vi "error.vi"(1 "error (in)":dbl, 2 "Meas":dbl, 3 "Req":dbl) -> (0 "error (out)":dbl)   [LabVIEW 2021]
panel:
  in  "k":dbl=1.0
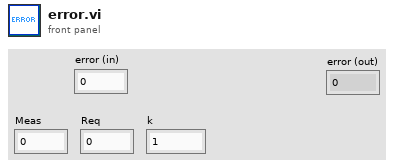
[diagram p1: front panel]
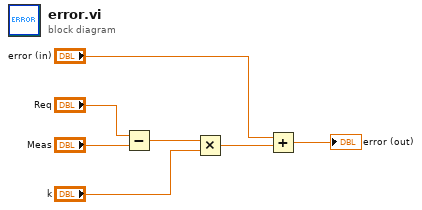
[diagram p0: block diagram]
diagram:
  n1 = Subtract(x="Req", y="Meas") -> (x-y=w7:dbl)
  n2 = Multiply(x=w7, y="k") -> (x*y=w5:dbl)
  n3 = Add(x="error (in)", y=w5) -> (x+y=→"error (out)":dbl)
